vi "zad3.vi"() -> ()   [LabVIEW 2017]
panel:
  out "Po zastosowaniu filtra":dynamicdata(graph)
  out "Przed zastosowaniem filtra":dynamicdata(graph)
  in  "Odciecie filtru":dbl
  in  "Czêstotliwoœæ próbkowania dzwieku":dbl
  in  "D³ugoœæ nagrywanego dzwieku w sekundach":dbl
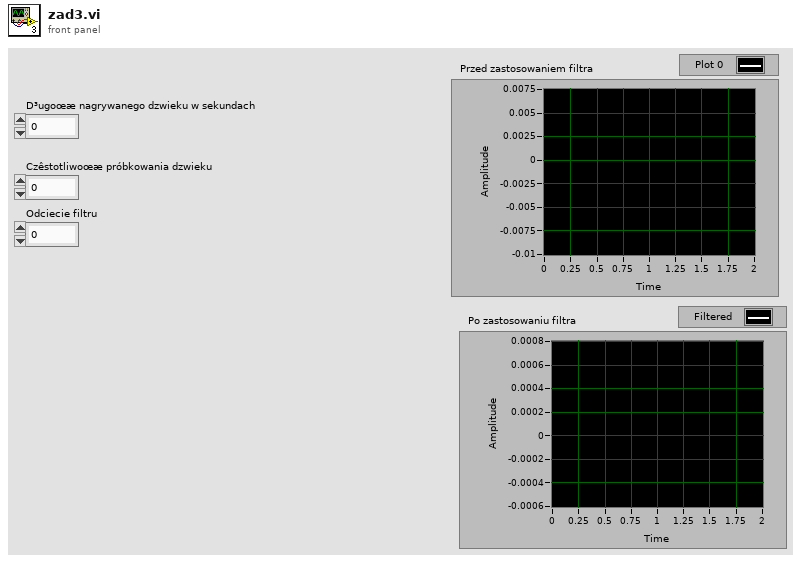
[diagram p1: front panel]
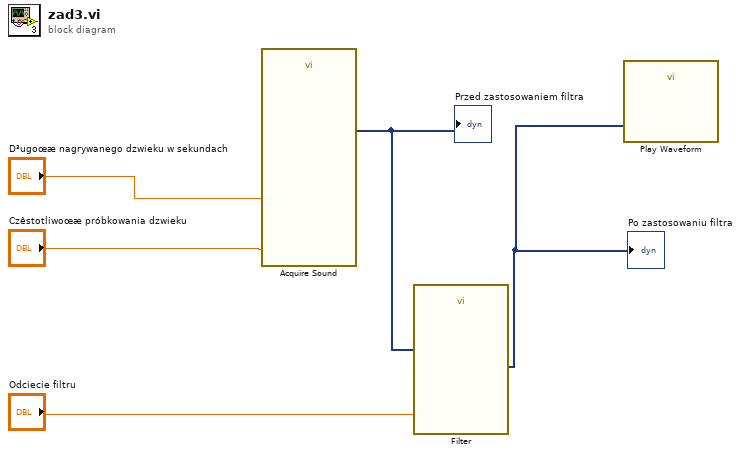
[diagram p0: block diagram]
diagram:
  n1 = call "Acquire Sound"("Duration (s)"="D³ugoœæ nagrywanego dzwieku w sekundach", "Sample rate (Hz)"="Czêstotliwoœæ próbkowania dzwieku") -> ("Data"=w1:dynamicdata)  [unwired: 16 in, 1 out]
  "Przed zastosowaniem filtra" <- w1
  n2 = call "Filter"("Lower Cut-Off"="Odciecie filtru", "Signal"=w1) -> ("Filtered Signal"=w2:dynamicdata)  [unwired: 8 in, 1 out]
  "Po zastosowaniu filtra" <- w2
  n3 = call "Play Waveform"("Data"=w2) -> ()  [unwired: 18 in, 1 out]
